vi "FringeScannerController.vi"() -> ()   [LabVIEW 2009]
uses:
  Nicmos/Controls/NICMOS.READOUT.ctl
  Controls/FringeScannerState.ctl
  Controls/FringeScannerCommand.ctl
  Controls/FringeScannerData.ctl
panel:
  out "State":T1
  out "OPD stroke":dbl[unit]
  out "READOUT":T2={"Readout"=100, "Deglitch"=10, "Framerate"=200.0, "Bank"=2}
  in  "PROCESS":string="FRINGESCANNER"
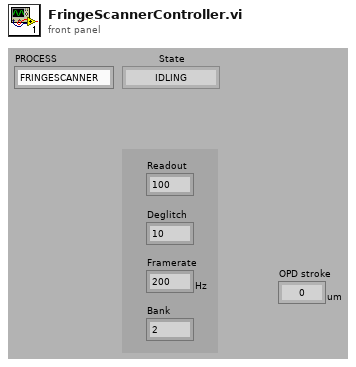
[diagram p1: front panel]
types:
  T1 = typedef "FringeScannerState.ctl" = enum16{"IDLING", "CONFIGURING", "SCANNING", "STOPPING"}
  T2 = typedef "NICMOS.READOUT.ctl" = cluster{"Readout":i32, "Deglitch":i32, "Framerate":dbl[unit], "Bank":i32}
  T3 = typedef "FringeScannerData.ctl" = cluster{"Readout":T2, "Wavelength":dbl[unit], "Frame per fringe":dbl, "Autcollimation":bool}
  T4 = typedef "FringeScannerCommand.ctl" = cluster{"Command":enum16{"IDLE", "SCAN", "QUIT"}, "FringeScannerData":T3}
  T5 = typedef "FringeTrackerSynchro.ctl" = cluster{"Command":refnum<queue>, "State":refnum<notifier>}
  T6 = typedef "PIEZO.WAVE.ctl" = cluster{"Speed":dbl[unit], "Stiffness (0.95)":dbl, "Linear Stroke":dbl[unit], "Delay":dbl[unit]}
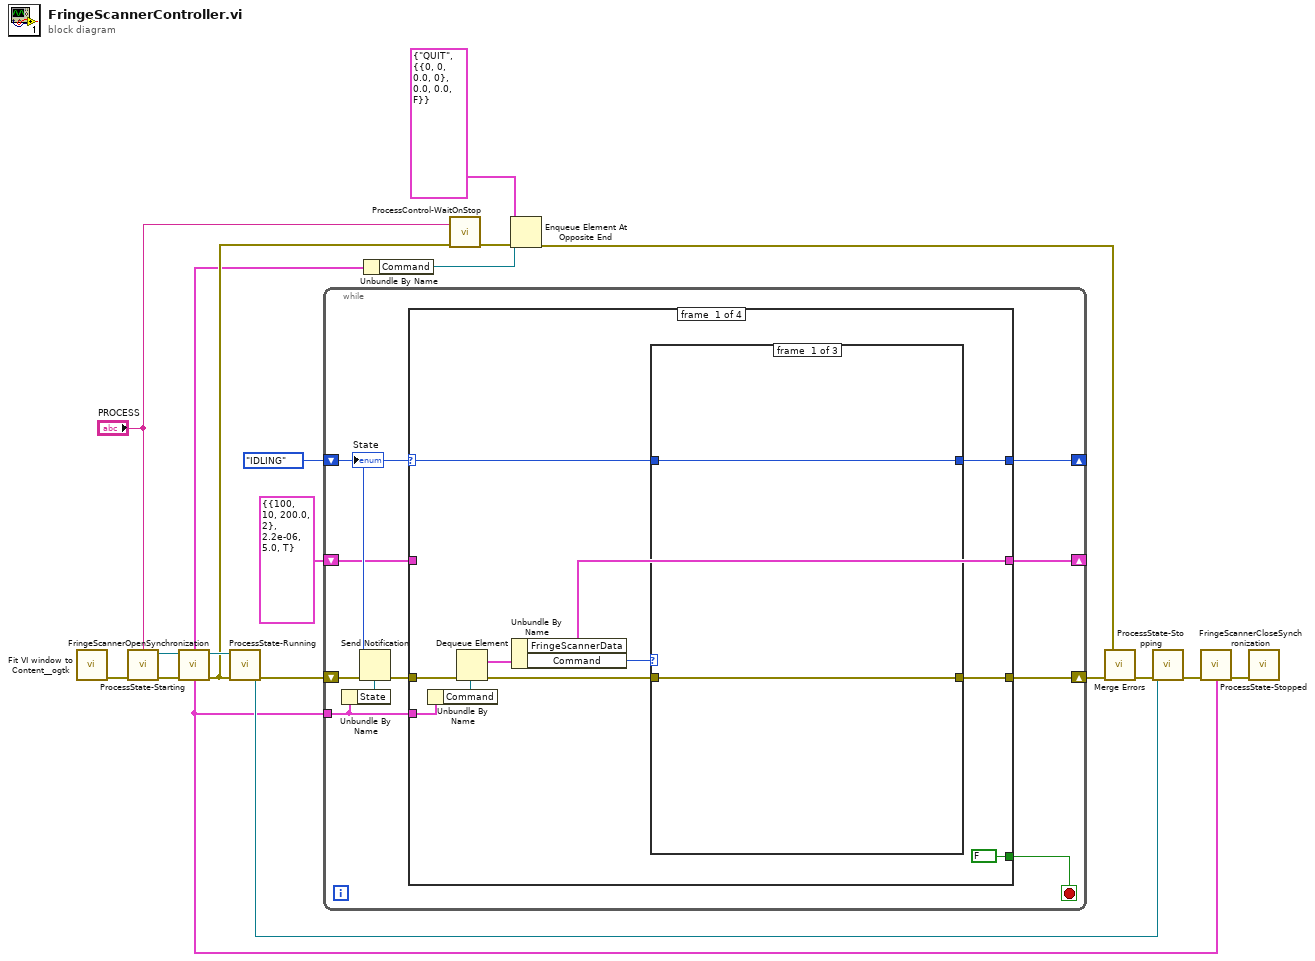
[diagram p0: block diagram]
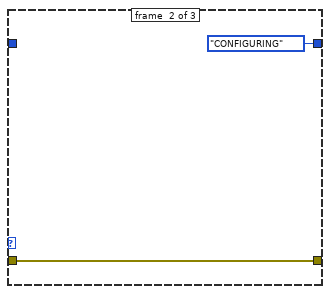
[diagram p2: hidden frame]
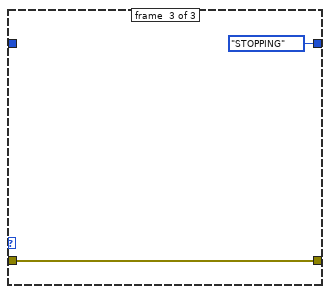
[diagram p3: hidden frame]
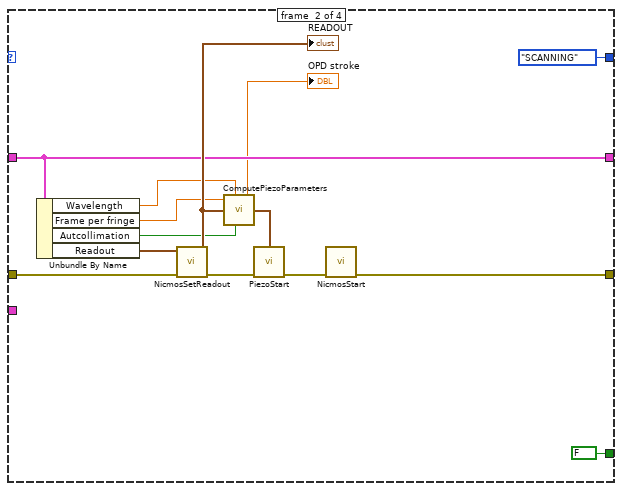
[diagram p4: hidden frame]
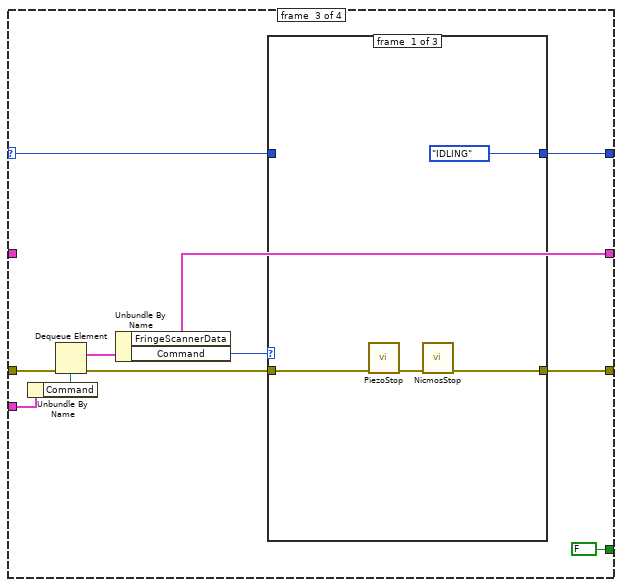
[diagram p5: hidden frame]
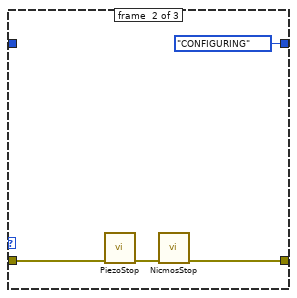
[diagram p6: hidden frame]
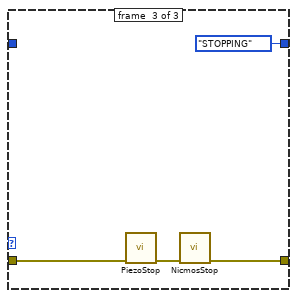
[diagram p7: hidden frame]
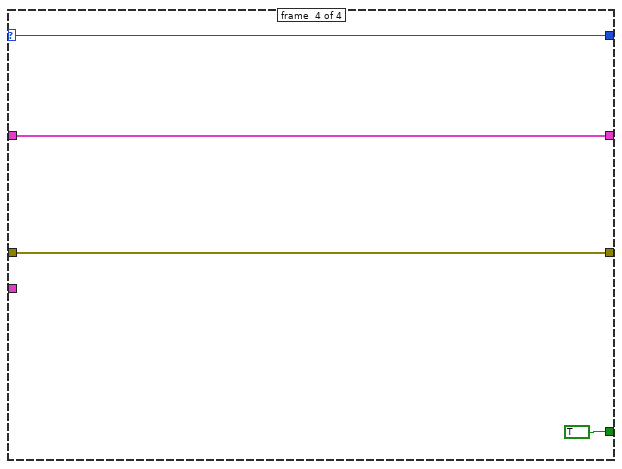
[diagram p8: hidden frame]
diagram:
  n1 = call <userlib>:"Fit VI window to Content__ogtk.vi"() -> ("error out"=w18:errorcluster)  [unwired: 6 in, 1 out]
  n2 = call "ProcessState-Starting.vi"("PROCESS"="PROCESS", "error in (no error)"=w18) -> ("ProcessStateNotifier"=w14:refnum<notifier>, "error in (no error)"=w16:errorcluster)  [unwired: 6 in]
  n3 = call "FringeScannerOpenSynchronization.vi"("error in (no error)"=w16) -> ("FringeTrackerSynchro"=w2:T5, "error out"=w13:errorcluster)  [unwired: 7 in]
  n4 = call "ProcessState-Running.vi"("ProcessStateNotifier in"=w14, "error in (no error)"=w13) -> ("ProcessStateNotifier out"=w5:refnum<notifier>, "error out"=w15:errorcluster)  [unwired: 6 in]
  n5 = while {
    shift-right: [w23] -> w8
    shift-left: w15 -> [w28]
    shift-right: [w22] -> _
    shift-left: FringeScannerState."IDLING" ("FringeScannerState") -> [w25]
    tunnel: w2 -> [w24]
    shift-right: [w20] -> _
    shift-left: T3 {"Readout"={"Readout"=100, "Deglitch"=10, "Framerate"=200.0, "Bank"=2}, "Wavelength"=2.2e-06, "Frame per fringe"=5.0, "Autcollimation"=TRUE} ("FringeScannerData") -> [w19]
    stop <- w21 stop-if-true
    n6 = Unbundle By Name(w24) -> ("State"=w26:refnum<notifier>)
    n7 = Send Notification(notification=w25, notifier=w26, error in (no error)=w28) -> (error out=w27:errorcluster)  [unwired: 1 out]
    n8 = case shown="\"CONFIGURING\"" w25 {
      selector: w25 -> [w34 _ w65 w86]
      tunnel: w27 -> [w38 w56 w69 w85]
      tunnel: w24 -> [w39 _ w70 _]
      tunnel: [w35 w55 w66 w85] -> w23
      tunnel: [w33 FringeScannerState."SCANNING" ("FringeScannerState") w64 w86] -> w22
      tunnel: [FALSE FALSE FALSE TRUE] -> w21
      tunnel: [w29 w47 w60 w83] -> w20
      tunnel: w19 -> [_ w47 _ w83]
      frame #0 {
        n9 = Unbundle By Name(w39) -> ("Command"=w37:refnum<queue>)
        n10 = Dequeue Element(queue=w37, error in (no error)=w38) -> (element=w30:T4, error out=w36:errorcluster)  [unwired: 1 in, 2 out]
        n11 = Unbundle By Name(w30) -> ("FringeScannerData"=w29:T3, "Command"=w31:enum16{"IDLE", "SCAN", "QUIT"})
        n12 = case shown="\"IDLE\", Default" w31 {
          tunnel: w36 -> [w41 w42 w44]
          tunnel: [w41 w42 w44] -> w35
          tunnel: w34 -> [w40 _ _]
          tunnel: [w40 FringeScannerState."CONFIGURING" ("FringeScannerState") FringeScannerState."STOPPING" ("FringeScannerState")] -> w33
          frame #0 {
          }
          frame #1 {
          }
          frame #2 {
          }
        }
      }
      frame #1 {
        n13 = Unbundle By Name(w47) -> ("Wavelength"=w48:dbl[unit], "Frame per fringe"=w49:dbl, "Autcollimation"=w50:bool, "Readout"=w51:T2)
        n14 = call "NicmosSetReadout.vi"("READOUT in"=w51, "error in (no error)"=w56) -> ("READOUT out"=w52:T2, "error out"=w59:errorcluster)  [unwired: 6 in]
        "READOUT" <- w52
        n15 = call "ComputePiezoParameters.vi"("Frame per fringe"=w49, "Wavelength"=w48, "READOUT"=w52, "Autcollimation"=w50) -> ("OPD stroke"=→"OPD stroke":dbl[unit], "WAVE"=w57:T6)  [unwired: 2 in]
        n16 = call "PiezoStart.vi"("WAVE"=w57, "error in (no error)"=w59) -> ("error out"=w58:errorcluster)  [unwired: 7 in]
        n17 = call "NicmosStart.vi"("error in (no error)"=w58) -> ("error out"=w55:errorcluster)  [unwired: 8 in]
      }
      frame #2 {
        n18 = Unbundle By Name(w70) -> ("Command"=w68:refnum<queue>)
        n19 = Dequeue Element(queue=w68, error in (no error)=w69) -> (element=w61:T4, error out=w67:errorcluster)  [unwired: 1 in, 2 out]
        n20 = Unbundle By Name(w61) -> ("FringeScannerData"=w60:T3, "Command"=w62:enum16{"IDLE", "SCAN", "QUIT"})
        n21 = case shown="\"SCAN\"" w62 {
          tunnel: w67 -> [w74 w77 w81]
          tunnel: [w72 w76 w80] -> w66
          tunnel: w65 -> [_ _ _]
          tunnel: [FringeScannerState."IDLING" ("FringeScannerState") FringeScannerState."CONFIGURING" ("FringeScannerState") FringeScannerState."STOPPING" ("FringeScannerState")] -> w64
          frame #0 {
            n22 = call "PiezoStop.vi"("error in (no error)"=w74) -> ("error out"=w73:errorcluster)  [unwired: 10 in]
            n23 = call "NicmosStop.vi"("error in (no error)"=w73) -> ("error out"=w72:errorcluster)  [unwired: 8 in]
          }
          frame #1 {
            n24 = call "PiezoStop.vi"("error in (no error)"=w77) -> ("error out"=w78:errorcluster)  [unwired: 10 in]
            n25 = call "NicmosStop.vi"("error in (no error)"=w78) -> ("error out"=w76:errorcluster)  [unwired: 8 in]
          }
          frame #2 {
            n26 = call "PiezoStop.vi"("error in (no error)"=w81) -> ("error out"=w82:errorcluster)  [unwired: 10 in]
            n27 = call "NicmosStop.vi"("error in (no error)"=w82) -> ("error out"=w80:errorcluster)  [unwired: 8 in]
          }
        }
      }
      frame #3 {
      }
    }
    "State" <- w25
  }
  n28 = Unbundle By Name(w2) -> ("Command"=w10:refnum<queue>)
  n29 = call "ProcessControl-WaitOnStop.vi"("PROCESS"="PROCESS", "error out"=w13) -> ("error in"=w11:errorcluster)  [unwired: 7 in]
  n30 = Enqueue Element At Opposite End(queue=w10, element=T4 {"Command"=enum."QUIT", "FringeScannerData"={"Readout"={"Readout"=0, "Deglitch"=0, "Framerate"=0.0, "Bank"=0}, "Wavelength"=0.0, "Frame per fringe"=0.0, "Autcollimation"=FALSE}}, error in (no error)=w11) -> (error out=w7:errorcluster)  [unwired: 1 in, 2 out]
  n31 = call <vilib>:"Merge Errors.vi"("error in 3 (no error)"=w8, "error in 1 (no error)"=w7) -> ("error out"=w6:errorcluster)  [unwired: 5 in]
  n32 = call "ProcessState-Stopping.vi"("ProcessStateNotifier in"=w5, "error in (no error)"=w6) -> ("error out"=w4:errorcluster)  [unwired: 6 in, 1 out]
  n33 = call "FringeScannerCloseSynchronization.vi"("FringeTrackerSynchro"=w2, "error in (no error)"=w4) -> ("error out"=w3:errorcluster)  [unwired: 7 in]
  n34 = call "ProcessState-Stopped.vi"("error in (no error)"=w3) -> ()  [unwired: 8 in, 1 out]
